vi "Generate Trace.vi"(11 "String":string) -> ()   [LabVIEW 2020, in "Actor Framework.lvlib"]
uses:
  Actor Framework.lvlib
  Inspection API/AF Trace Format/AF Trace Format.lvclass
  <resource>/dialog/lvconfig.llb/LV Config Read String.vi
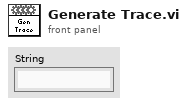
[diagram p1: front panel]
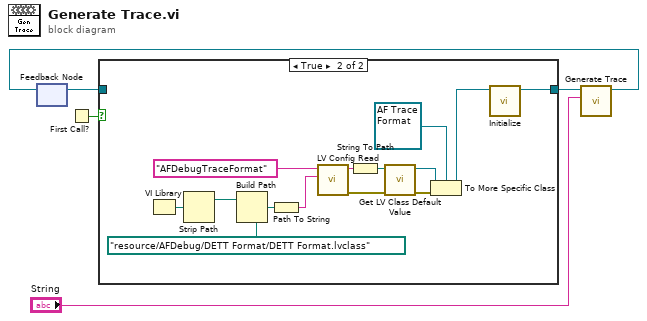
[diagram p0: block diagram]
diagram:
  n1 = feedback #1() -> (w4:refnum<class "AF Trace Format.lvclass">)  [unwired: 1 in]
  n2 = First Call?() -> (First Call?: T/F=w1:bool)
  n3 = case shown="True" w1 {
    tunnel: w4 -> [w6 _]
    tunnel: [w6 w8] -> w3
    frame False {
    }
    frame True {
      n4 = VI Library() -> (path=w19:path)
      n5 = Strip Path(path=w19) -> (stripped path=w18:path)  [unwired: 1 out]
      n6 = Build Path(base path=w18, name or relative path=path "resource/AFDebug/DETT Format/DETT Format.lvclass") -> (appended path=w16:path)
      n7 = Path To String(path=w16) -> (string=w15:string)
      n8 = call-poly <resource>:"LV Config Read.vi"("default value"=w15, "key"="AFDebugTraceFormat") -> ("error out"=w14:errorcluster, "value"=w12:string)  [unwired: 3 in, 1 out]
      n9 = String To Path(string=w12) -> (path=w13:path)
      n10 = call <vilib>:"Get LV Class Default Value.vi"("error in (no error)"=w14, "class path"=w13) -> ("error out"=w11:errorcluster, "object"=w10:refnum<class>)  [unwired: 8 in]
      n11 = To More Specific Class(target class=refnum<class "AF Trace Format.lvclass"> refnum ("Actor Framework:AF Trace Format.lvclass"), reference=w10, error in=w11) -> (specific class reference=w9:refnum<class "AF Trace Format.lvclass">)  [unwired: 1 out]
      n12 = call-dynamic "Initialize.vi"("AF Trace Format in"=w9) -> ("AF Trace Format out"=w8:refnum<class "AF Trace Format.lvclass">)  [unwired: 9 in, 1 out]
    }
  }
  n13 = call-dynamic "Generate Trace.vi"("Trace String"="String", "AF Trace Format in"=w3) -> ("AF Trace Format out"=w2:refnum<class "AF Trace Format.lvclass">)  [unwired: 9 in]
  n14 = feedback-in #1(w2) -> ()
